vi "Close.vi"(8 "error in (no error)":errorcluster, 11 "BaseResponder in":refnum<class "BaseResponder.lvclass">) -> (0 "error out":errorcluster, 3 "BaseResponder out":refnum<class "BaseResponder.lvclass">)   [LabVIEW 2013, in "BaseResponder.lvclass"]
doc: "Closes all open references and reserved resources for the responder"
uses:
  BaseResponder.lvclass
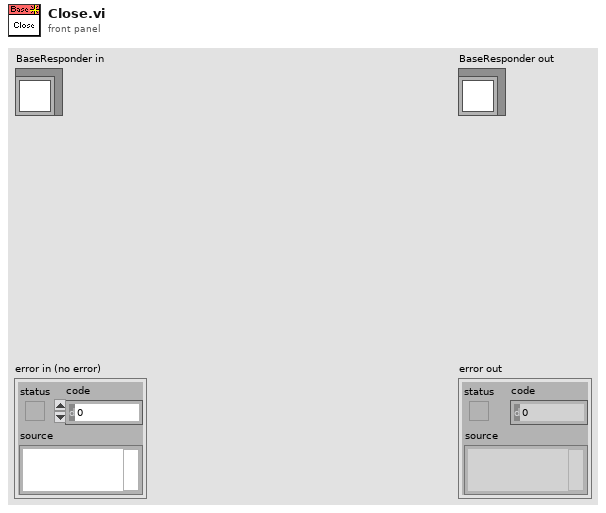
[diagram p1: front panel]
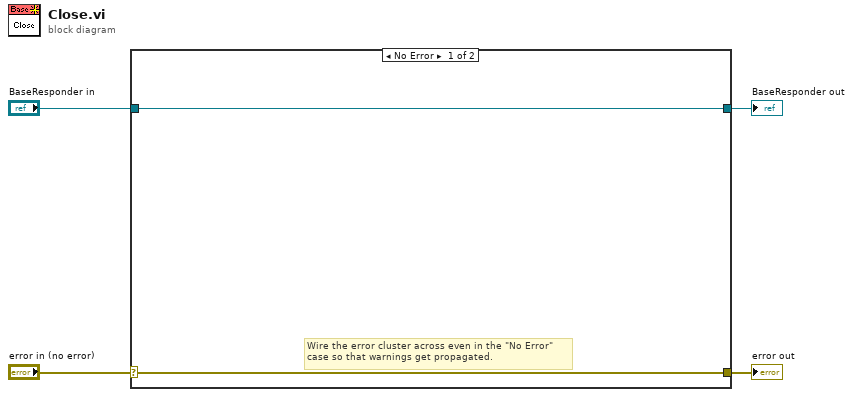
[diagram p0: block diagram]
diagram:
  n1 = case shown="No Error" "error in (no error)" {
    selector: "error in (no error)" -> [w5 w8]
    tunnel: [w5 w8] -> w3
    tunnel: [w6 w7] -> w1
    tunnel: "BaseResponder in" -> [w6 w7]
    frame No Error {
      # "Wire the error cluster across even in the \"No Error\"\ncase so that warnings get propagated."
    }
    frame Error {
    }
  }
  "error out" <- w3
  "BaseResponder out" <- w1
